vi "To Standard Sequence.vi"(8 "error in (no error)":errorcluster, 11 "Sequence Config in":refnum<class "Sequence Config.lvclass">) -> (0 "error out":errorcluster, 2 "Standard Sequence":string[][](array[string])=[["Simple", "", "", ""], ["Wait", "1000", "", ""], ["Update", "Boolean result 0", "Boolean", "True"], ["Wait ", "1000", "", ""], ["Update", "Boolean result 0", "Boolean", "False"]], 3 "Sequence Config out":refnum<class "Sequence Config.lvclass">)   [LabVIEW 2015, in "Sequence Config.lvclass"]
uses:
  Sequence Config.lvclass
  Step/Config/Step Config.lvclass
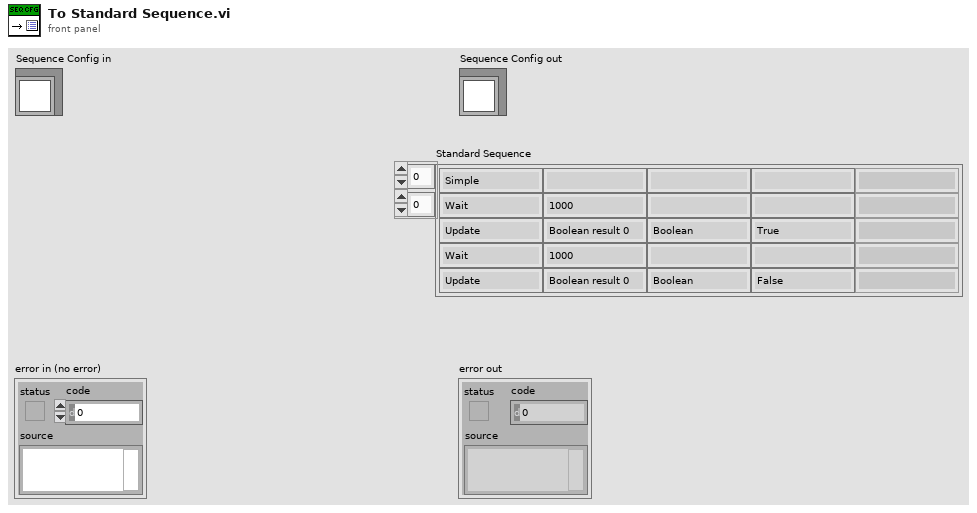
[diagram p1: front panel]
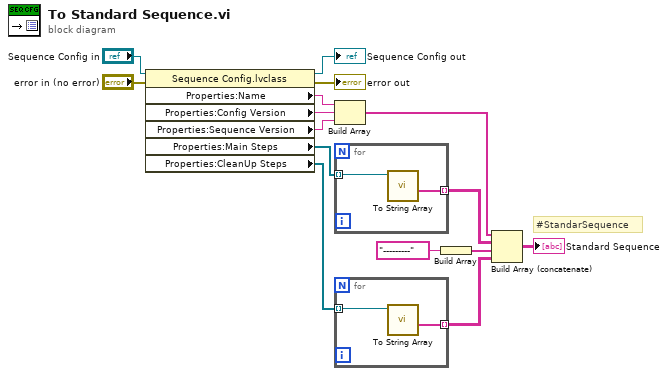
[diagram p0: block diagram]
diagram:
  # "#StandarSequence"
  n1 = property class="Sequence Config.lvclass"(reference="Sequence Config in", error in="error in (no error)") -> (reference out=→"Sequence Config out":refnum<class "Sequence Config.lvclass">, error out=→"error out":errorcluster, "Properties:Name"=w1:string, "Properties:Config Version"=w2:string, "Properties:Sequence Version"=w3:string, "Properties:Main Steps"=w4:refnum<class "Step Config.lvclass">[], "Properties:CleanUp Steps "=w5:refnum<class "Step Config.lvclass">[])
  n2 = Build Array(w1, w2, w3) -> (w15:string[])
  n3 = for {
    tunnel: w4 -> [w17] mode=indexing
    tunnel: [w16] -> w14 mode=indexing
    n4 = call-dynamic "To String Array.vi"("Step Config in"=w17) -> ("Step String Array"=w16:string[])  [unwired: 8 in, 2 out]
  }
  n5 = for {
    tunnel: w5 -> [w19] mode=indexing
    tunnel: [w18] -> w12 mode=indexing
    n6 = call-dynamic "To String Array.vi"("Step Config in"=w19) -> ("Step String Array"=w18:string[])  [unwired: 8 in, 2 out]
  }
  n7 = Build Array("---------") -> (w10:string[])
  n8 = Build Array (concatenate)(w15, w14, w10, w12) -> (→"Standard Sequence":string[][])
